vi "Find Circle Grade.vi"(9 "Picture":u8[][](array[numeric]), 10 "Cluster":T1) -> (0 "MaxX":u32, 1 "MaxY":u32, 2 "MaxA":u32, 3 "MaxGrade":u32, 4 "MaxB":u32)   [LabVIEW 2015]
uses:
  Controls/Pivot Finder Input Params Typedef.ctl
panel:
  out "Picture 2":u8[][](graph)
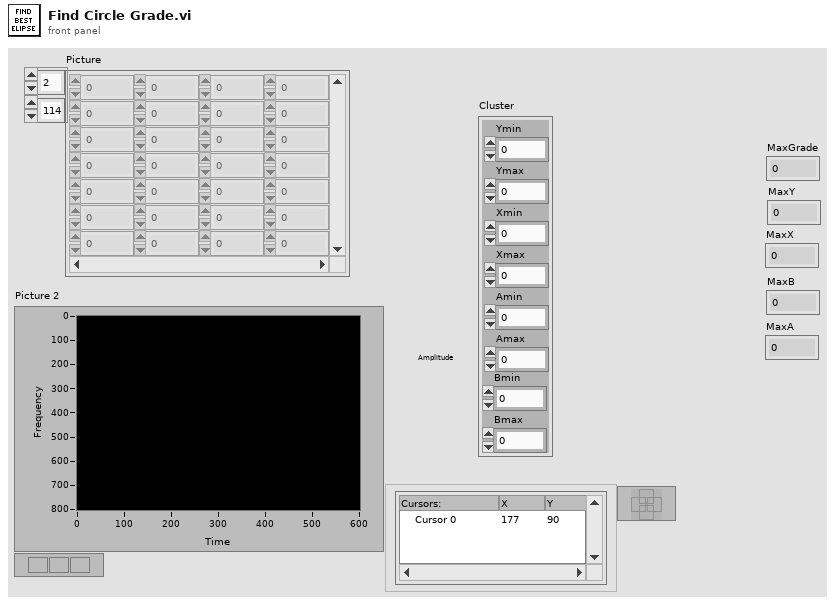
[diagram p1: front panel]
types:
  T1 = typedef "Pivot Finder Input Params Typedef.ctl" = cluster{"Ymin":u32, "Ymax":u32, "Xmin":u32, "Xmax":u32, "Amin":u32, "Amax":u32, "Bmin":u32, "Bmax":u32}
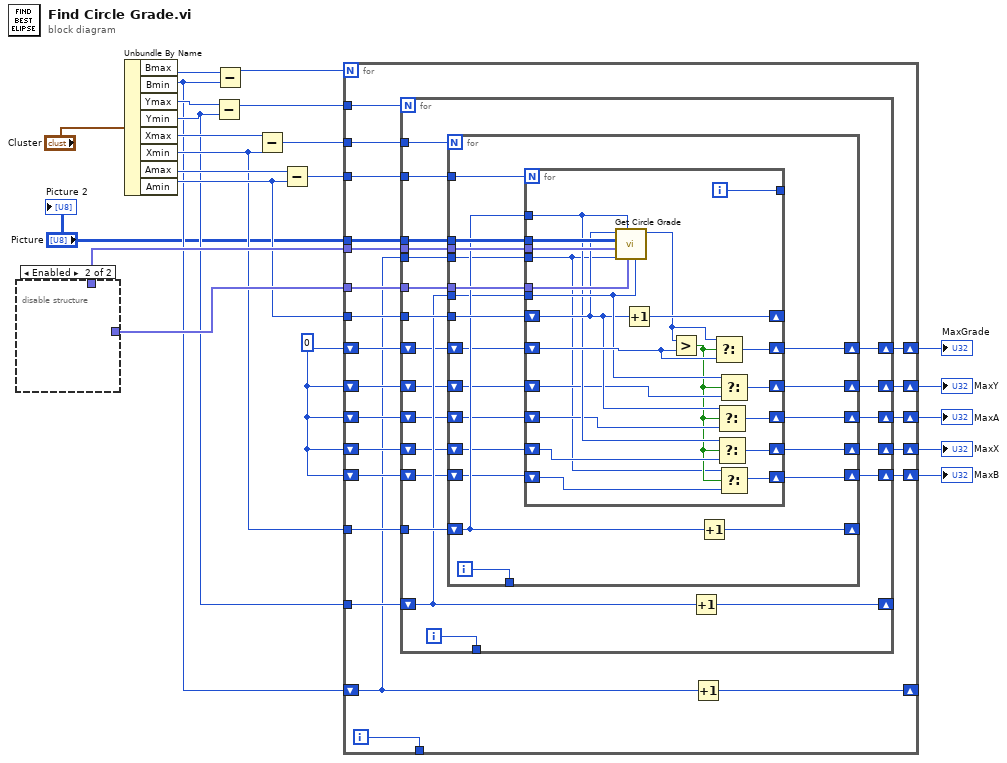
[diagram p0: block diagram]
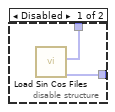
[diagram p2: hidden frame]
diagram:
  w7 = u32 0 ("Grade")
  n1 = disable-structure shown="Enabled" {
    disable-tunnel: [w24 _] -> w22
    disable-tunnel: [w23 _] -> w21
    frame Disabled {
      n2 = call "Load Sin Cos Files.vi"() -> ("Sin Fixed"=w23:fxp<+/-,32,1>[], "Cos Fixed"=w24:fxp<+/-,32,1>[])  [unwired: 8 in, 2 out]
    }
    frame Enabled {
    }
  }
  n3 = Unbundle By Name("Cluster") -> ("Bmax"=w4:u32, "Bmin"=w2:u32, "Ymax"=w19:u32, "Ymin"=w12:u32, "Xmax"=w18:u32, "Xmin"=w13:u32, "Amax"=w17:u32, "Amin"=w15:u32)
  n4 = Subtract(x=w19, y=w12) -> (x-y=w6:u32)
  n5 = Subtract(x=w4, y=w2) -> (x-y=w5:u32)
  n6 = Subtract(x=w18, y=w13) -> (x-y=w14:u32)
  n7 = Subtract(x=w17, y=w15) -> (x-y=w16:u32)
  n8 = for {
    N: w5 -> [_]
    tunnel: w22 -> [w46]
    tunnel: w21 -> [w45]
    tunnel: "Picture" -> [w44]
    tunnel: w16 -> [w43]
    tunnel: w15 -> [w42]
    tunnel: w14 -> [w41]
    tunnel: w13 -> [w40]
    tunnel: w12 -> [w39]
    tunnel: w6 -> [w38]
    shift-right: [w37] -> w11
    shift-left: w7 -> [w33]
    shift-right: [w36] -> w10
    shift-left: w7 -> [w32]
    shift-right: [w35] -> w9
    shift-left: w7 -> [w31]
    shift-right: [w34] -> w8
    shift-left: w7 -> [w30]
    shift-right: [w27] -> w3
    shift-left: w7 -> [w29]
    shift-right: [w28] -> _
    shift-left: w2 -> [w26]
    tunnel: [w25] -> _
    i -> [w25]
    n9 = for {
      N: w38 -> [_]
      tunnel: w46 -> [w67]
      tunnel: w45 -> [w66]
      tunnel: w44 -> [w65]
      tunnel: w43 -> [w64]
      tunnel: w42 -> [w63]
      tunnel: w41 -> [w62]
      tunnel: w40 -> [w61]
      shift-right: [w60] -> _
      shift-left: w39 -> [w59]
      shift-right: [w57] -> w37
      shift-left: w33 -> [w58]
      shift-right: [w56] -> w36
      shift-left: w32 -> [w53]
      shift-right: [w55] -> w35
      shift-left: w31 -> [w52]
      shift-right: [w54] -> w34
      shift-left: w30 -> [w51]
      shift-right: [w49] -> w27
      shift-left: w29 -> [w50]
      tunnel: w26 -> [w48]
      tunnel: [w47] -> _
      i -> [w47]
      n10 = for {
        N: w62 -> [_]
        tunnel: w67 -> [w87]
        tunnel: w66 -> [w86]
        tunnel: w65 -> [w85]
        tunnel: w64 -> [w84]
        tunnel: w63 -> [w83]
        shift-right: [w82] -> _
        shift-left: w61 -> [w81]
        tunnel: w59 -> [w80]
        shift-right: [w78] -> w57
        shift-left: w58 -> [w79]
        shift-right: [w77] -> w56
        shift-left: w53 -> [w74]
        shift-right: [w76] -> w55
        shift-left: w52 -> [w73]
        shift-right: [w75] -> w54
        shift-left: w51 -> [w72]
        shift-right: [w70] -> w49
        shift-left: w50 -> [w71]
        tunnel: w48 -> [w69]
        tunnel: [w68] -> _
        i -> [w68]
        n11 = for {
          N: w84 -> [_]
          tunnel: w87 -> [w108]
          tunnel: w86 -> [w107]
          tunnel: w85 -> [w106]
          shift-right: [w105] -> _
          shift-left: w83 -> [w100]
          tunnel: w81 -> [w99]
          tunnel: w80 -> [w101]
          shift-right: [w102] -> w78
          shift-left: w79 -> [w103]
          shift-right: [w95] -> w77
          shift-left: w74 -> [w96]
          shift-right: [w94] -> w76
          shift-left: w73 -> [w97]
          shift-right: [w93] -> w75
          shift-left: w72 -> [w98]
          shift-right: [w92] -> w70
          shift-left: w71 -> [w91]
          tunnel: w69 -> [w89]
          tunnel: [w88] -> _
          i -> [w88]
          n12 = call "Get Circle Grade.vi"("Y"=w101, "Sin Fixed"=w107, "X"=w99, "B"=w89, "Cos Fixed"=w108, "Picture"=w106, "A"=w100) -> ("Grade"=w104:u32)  [unwired: 4 in]
          n13 = Increment(x=w100) -> (x+1=w105:u32)
          n14 = Greater?(x=w104, y=w103) -> (0:w90:bool)
          n15 = Select(t=w104, s=w90, f=w103) -> (s? t:f=w102:u32)
          n16 = Select(t=w100, s=w90, f=w97) -> (s? t:f=w94:u32)
          n17 = Select(t=w99, s=w90, f=w98) -> (s? t:f=w93:u32)
          n18 = Select(t=w101, s=w90, f=w96) -> (s? t:f=w95:u32)
          n19 = Select(t=w89, s=w90, f=w91) -> (s? t:f=w92:u32)
        }
        n20 = Increment(x=w81) -> (x+1=w82:u32)
      }
      n21 = Increment(x=w59) -> (x+1=w60:u32)
    }
    n22 = Increment(x=w26) -> (x+1=w28:u32)
  }
  "MaxGrade" <- w11
  "MaxY" <- w10
  "MaxA" <- w9
  "MaxX" <- w8
  "MaxB" <- w3
  "Picture 2" <- "Picture"
